vi "Ejercicio 3.2.vi"() -> ()   [LabVIEW 2020]
uses:
  <vilib>/numeric/Random Number (Range) DBL.vi
panel:
  out "Dato final":dbl
  out "Valor máximo señal 2":dbl
  out "Valor máximo señal 1":dbl
  out "Ejercicio 3.2":dynamicdata(graph)
  out "Señal 2":dbl[](array[numeric])
  out "Señal 1":dbl[](array[numeric])
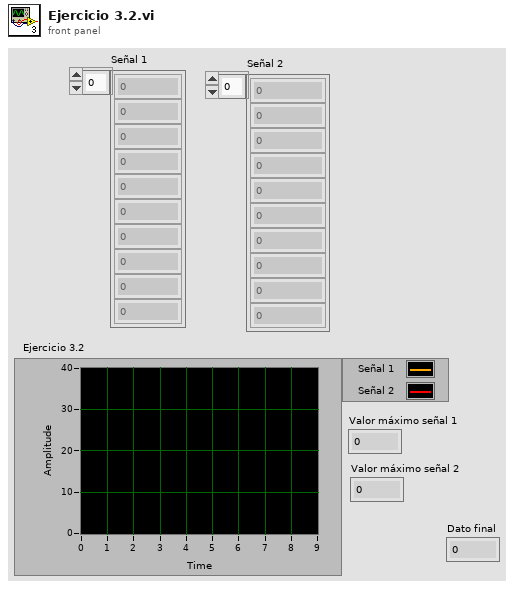
[diagram p1: front panel]
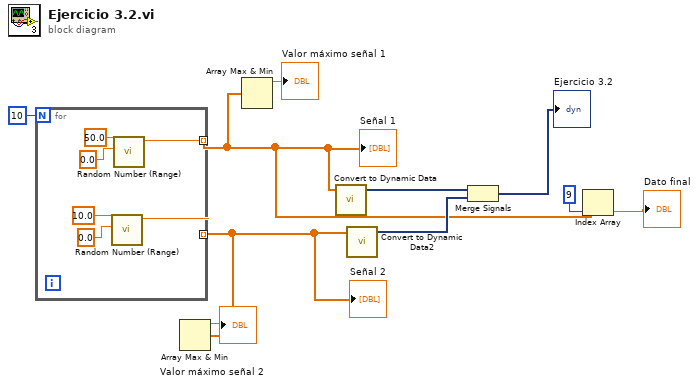
[diagram p0: block diagram]
diagram:
  n1 = for {
    N: 10 -> [_]
    tunnel: [w14] -> w4 mode=indexing
    tunnel: [w11] -> w1 mode=indexing
    n2 = call-poly <vilib>:"Random Number (Range).vi"("lower bound (0)"=0.0, "upper bound (100)"=10.0) -> ("number"=w11:dbl)  [unwired: 9 in]
    n3 = call-poly <vilib>:"Random Number (Range).vi"("lower bound (0)"=0.0, "upper bound (100)"=50.0) -> ("number"=w14:dbl)  [unwired: 9 in]
  }
  "Señal 1" <- w4
  "Señal 2" <- w1
  n4 = Array Max & Min(array=w1) -> (max value=→"Valor máximo señal 2":dbl)  [unwired: 3 out]
  n5 = Array Max & Min(array=w4) -> (max value=→"Valor máximo señal 1":dbl)  [unwired: 3 out]
  n6 = call "Convert to Dynamic Data"("Array"=w4) -> ("Dynamic Data Type"=w9:dynamicdata)  [unwired: 3 in]
  n7 = call "Convert to Dynamic Data2"("Array"=w1) -> ("Dynamic Data Type"=w8:dynamicdata)  [unwired: 3 in]
  n8 = Merge Signals "Merge Signals"(w9, w8) -> (→"Ejercicio 3.2":dynamicdata)
  n9 = Index Array(array=w4, index=9) -> (element=→"Dato final":dbl)
